vi "ROS_Master_GetSubInfo.vi"(1 "Direction":enum16{"Publisher", "Subscriber"}(ring)=enum."Subscriber", 2 "String w/o Tag":string) -> (0 "PubSub":T1)   [LabVIEW 2012]
doc: "Takes an XML string and returns a cluster of\n-Topic\n-Direction\n-IP\n-Caller ID\n-Message Type"
uses:
  <userlib>/ROS for LabVIEW Software/ROS/Code/ROS_Master/ROS_Topic.ctl
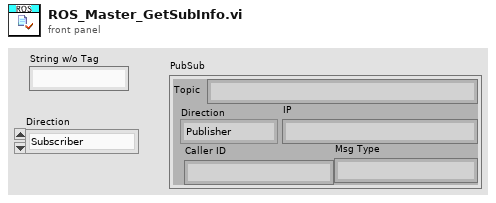
[diagram p1: front panel]
types:
  T1 = typedef "ROS_Topic.ctl" = cluster{"Caller ID":string, "IP":string, "Msg Type":string, "Direction":enum16{"Publisher", "Subscriber"}, "Topic":string}
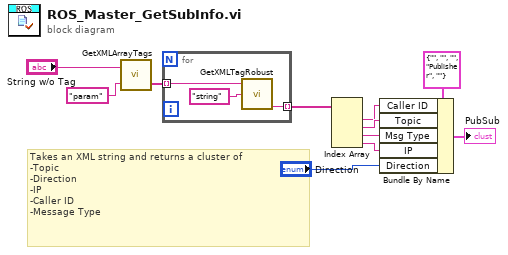
[diagram p0: block diagram]
diagram:
  # "Takes an XML string and returns a cluster of\n-Topic\n-Direction\n-IP\n-Caller ID\n-Message Type"
  n1 = call <userlib>:"GetXMLArrayTags.vi"("ArrayTag"="param", "String"="String w/o Tag") -> ("Array"=w3:string[])  [unwired: 1 out]
  n2 = for {
    tunnel: w3 -> [w14] mode=indexing
    tunnel: [w12] -> w4 mode=indexing
    n3 = call <userlib>:"GetXMLTagRobust.vi"("Tag"="string", "String"=w14) -> ("value"=w12:string)  [unwired: 1 in, 3 out]
  }
  n4 = Index Array(array=w4) -> (element #1=w5:string, element #2=w6:string, element #3=w7:string, element #4=w8:string)  [unwired: 4 in]
  n5 = Bundle By Name(cluster=T1 {"Caller ID"="", "IP"="", "Msg Type"="", "Direction"=enum."Publisher", "Topic"=""} ("PubSub"), "Caller ID"=w5, "Topic"=w6, "Msg Type"=w7, "IP"=w8, "Direction"="Direction") -> (→"PubSub":T1)
